vi "Features_SpecPage.vi"(10 "Spec Page Interface":T2, 11 "MetaDataObj in":refnum<class "MetaDataObj.lvclass">) -> (3 "MetaDataObj out":refnum<class "MetaDataObj.lvclass">)   [LabVIEW 2013, in "DCAFConfigurablePluginDecideFeatures.lvclass"]
uses:
  DCAFConfigurablePluginDecideFeatures.lvclass
  <resource>/dialog/NewProjectWizard/Spec Page Interface.ctl
  <resource>/dialog/NewProjectWizard/MetaDataObj/MetaDataObj.lvclass
  <vilib>/NI/Tag Bus/tag/Data Type.ctl
  <vilib>/NI/Tag Bus Module Framework/root configuration/Target Types.ctl
  <resource>/dialog/NewProjectWizard/MetaDataObj/MetaDataObj.lvclass/MetaDataObj.ctl
  DCAFConfigurablePluginDecideFeatures.lvclass/DCAFConfigurablePluginDecideFeatures.ctl
  <resource>/dialog/NewProjectWizard/MetaDataObj/Accessors/Write Project Name.vi
  Write component name.vi
  <resource>/dialog/NewProjectWizard/MetaDataObj/Accessors/Write Project Root.vi
  Write supported targets.vi
  Write supported data types.vi
  Write instances allowed.vi
  <resource>/dialog/NewProjectWizard/MetaDataObj/Accessors/Write File Prefix.vi
  <vilib>/NI/Tag Bus/tag/count types.vi
  <vilib>/NI/Tag Bus/tag/index to type.vi
  <vilib>/NI/Tag Bus Module Framework/root configuration/TBM configuration.lvclass
  <vilib>/NI/Tag Bus/tag/tag descriptor.lvclass
panel:
  in  "Tab Control":T1(tab)
  in  "Instances Allowed":i32=-1
  in  "Supported Targets":i32[](listbox)
  in  "Available Targets":i32[](listbox)
  in  "+target":bool
  in  "-target":bool
  in  "-type":bool
  in  "+type":bool
  in  "Available Data Types":i32[](listbox)
  in  "Supported Data Types":i32[](listbox)
  in  "Component Name":string
  in  "Project Root":path
  # "Execution Behaviors:"
  # "Number of classes allowed in a system. Default is infinite, -1. Examples: {PID: -1};{LED: 1}"
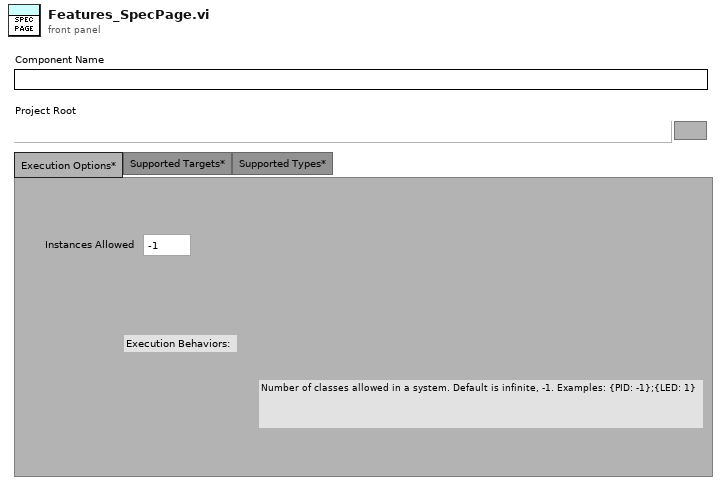
[diagram p1: front panel]
types:
  T1 = enum32{"Execution Options*", "Supported Targets*", "Supported Types*"}
  T2 = typedef "Spec Page Interface.ctl" = cluster{"\"Tab Forward To\" Refnum":refnum<vi>, "\"Tab Backward To\" Refnum":refnum<vi>, "Errors":refnum<user-event>, "Quit":refnum<user-event>}
  T3 = typedef "TBM configuration.lvclass/Target Types.ctl" = enum16{"Windows", "Mac", "Linux", "Linux RT ARM", "VxWorks", "Pharlap", "Other", "Linux RT x64"}
  T4 = typedef "tag bus.lvlib/tag descriptor.lvclass/Data Type.ctl" = enum16{"Double", "Single", "I64", "I32", "I16", "I8", "U64", "U32", "U16", "U8", "Boolean", "String", "Array of Double", "Array of Single", "Array of I64", "Array of I32", "Array of I16", "Array of I8", "Array of U64", "Array of U32", "Array of U16", "Array of U8", "Array of Boolean", "Array of String"}
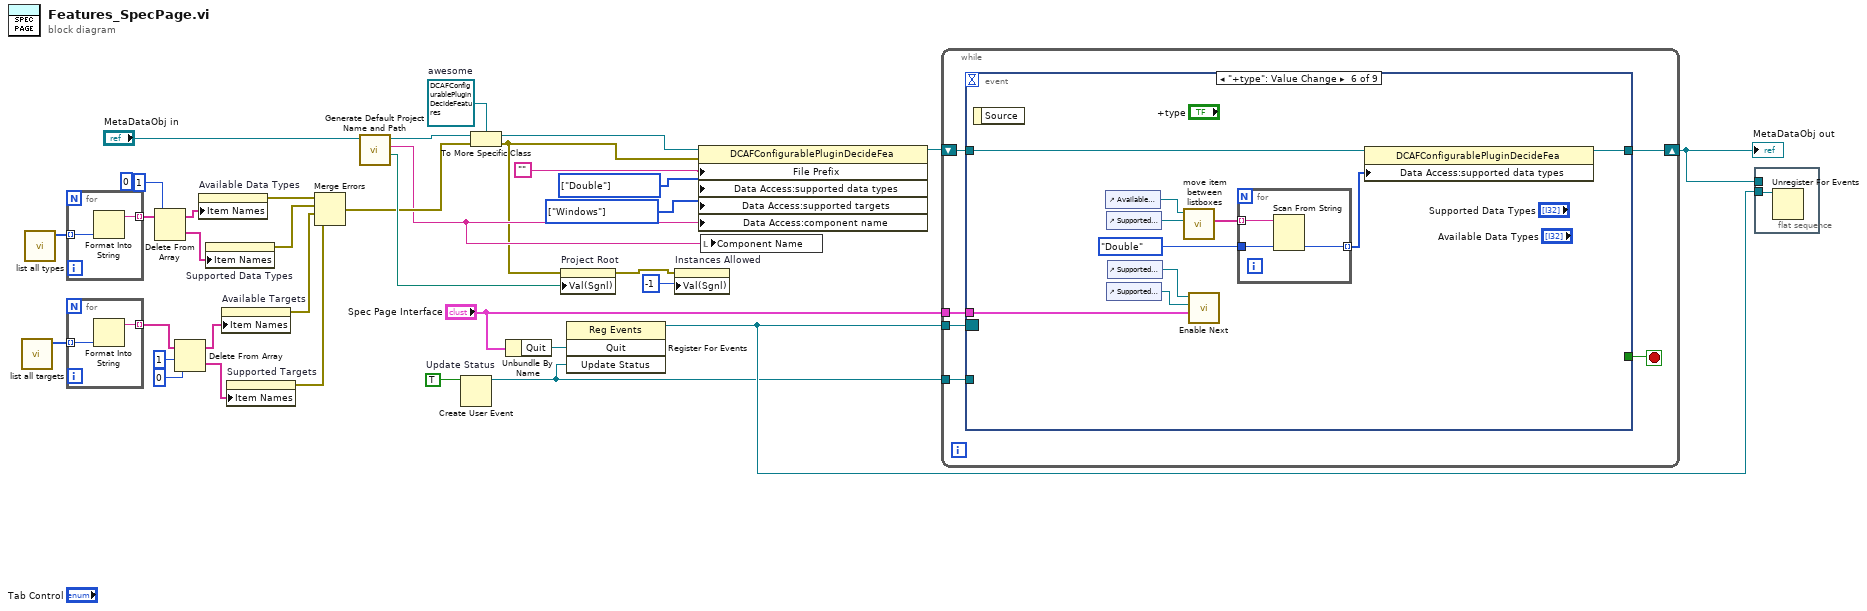
[diagram p0: block diagram]
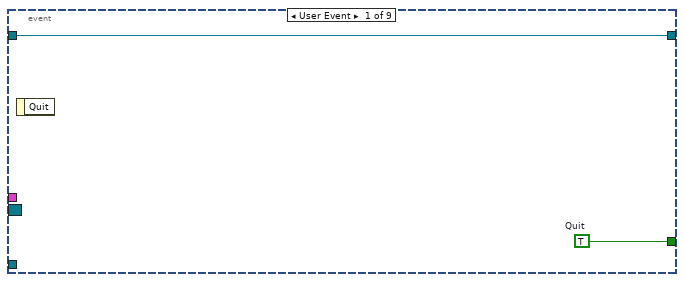
[diagram p2: hidden frame]
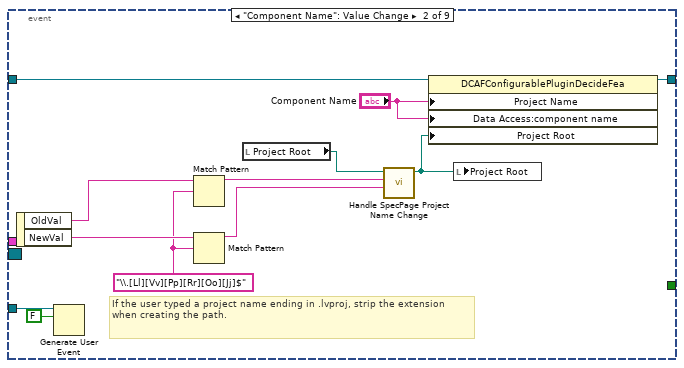
[diagram p3: hidden frame]
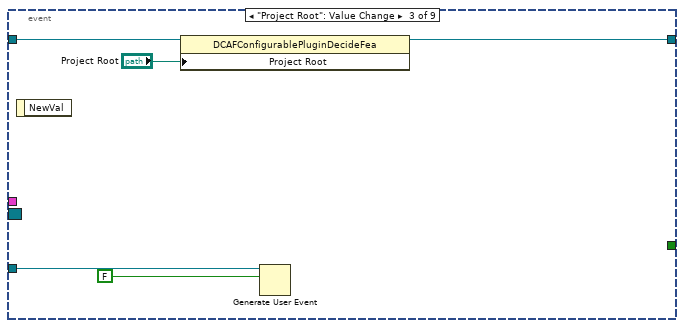
[diagram p4: hidden frame]
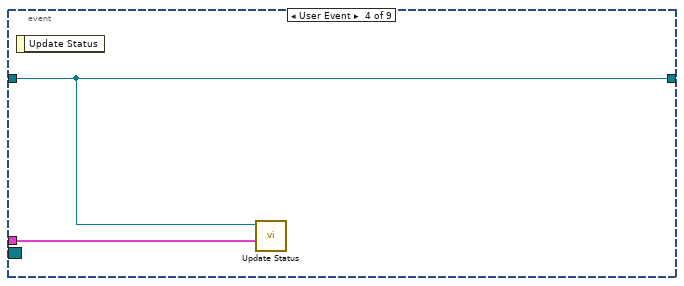
[diagram p5: hidden frame]
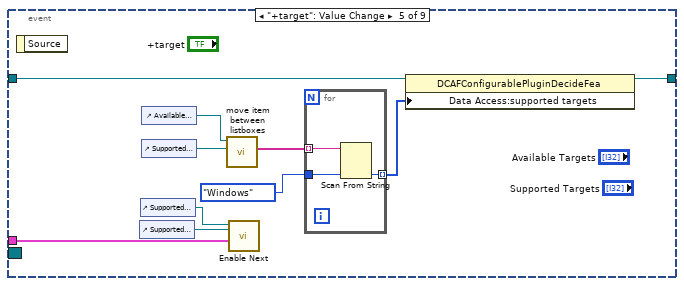
[diagram p6: hidden frame]
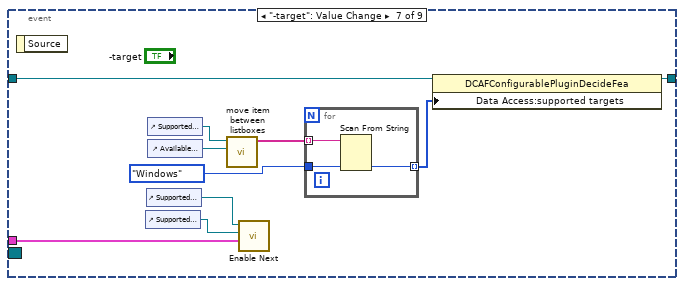
[diagram p7: hidden frame]
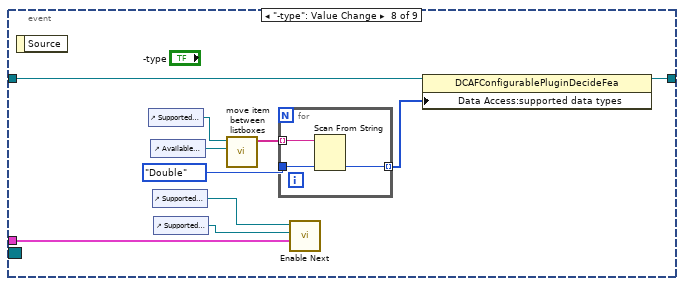
[diagram p8: hidden frame]
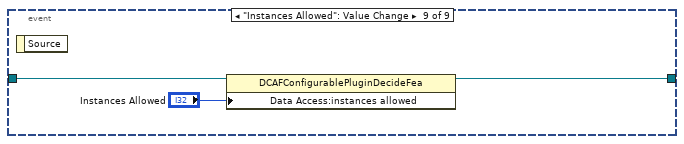
[diagram p9: hidden frame]
diagram:
  w1 = T3[] [enum."Windows"] items=["Windows", "Mac", "Linux", "Linux RT ARM", "VxWorks", "Pharlap", "Other", "Linux RT x64"] ("supported targets")
  w2 = T4[] [enum."Double"] items=["Double", "Single", "I64", "I32", "I16", "I8", "U64", "U32", "U16", "U8", "Boolean", "String", "Array of Double", "Array of Single", "Array of I64", "Array of I32", "Array of I16", "Array of I8", "Array of U64", "Array of U32", "Array of U16", "Array of U8", "Array of Boolean", "Array of String"] ("supported data types")
  w32 = TRUE  # Update Status
  w17 = refnum<class "DCAFConfigurablePluginDecideFeatures.lvclass"> refnum  # awesome
  n1 = call <vilib>:"list all targets.vi"() -> ("all targets"=w25:T3[])  [unwired: 11 in]
  n2 = call <vilib>:"list all types.vi"() -> ("all types"=w26:T4[])  [unwired: 11 in]
  n3 = for {
    tunnel: w26 -> [w38] mode=indexing
    tunnel: [w37] -> w16 mode=indexing
    n4 = Format Into String(w38) -> (resulting string=w37:string)  [unwired: 3 in, 1 out]
  }
  n5 = for {
    tunnel: w25 -> [w40] mode=indexing
    tunnel: [w39] -> w11 mode=indexing
    n6 = Format Into String(w40) -> (resulting string=w39:string)  [unwired: 3 in, 1 out]
  }
  n7 = Delete From Array(array=w16, length=1, index=0) -> (deleted portion=w14:string[], array with subset deleted=w15:string[])
  n8 = Delete From Array(array=w11, length=1, index=0) -> (deleted portion=w9:string[], array with subset deleted=w10:string[])
  n9 = property on="Available Data Types" class="LstBox (strict)"("Item Names"=w15) -> (error out=w24:errorcluster)  [unwired: 2 in, 1 out]
  n10 = property on="Supported Data Types" class="LstBox (strict)"("Item Names"=w14) -> (error out=w6:errorcluster)  [unwired: 2 in, 1 out]
  n11 = property on="Available Targets" class="LstBox (strict)"("Item Names"=w10) -> (error out=w23:errorcluster)  [unwired: 2 in, 1 out]
  n12 = property on="Supported Targets" class="LstBox (strict)"("Item Names"=w9) -> (error out=w5:errorcluster)  [unwired: 2 in, 1 out]
  n13 = Merge Errors(w24, w6, w23, w5) -> (w22:errorcluster)
  n14 = call <resource>:"Generate Default Project Name and Path.vi"("DNL_MetaDataObj in"="MetaDataObj in") -> ("Project Root"=w27:path, "Project Name"=w20:string, "DNL_MetaDataObj out"=w28:refnum<class "MetaDataObj.lvclass">)  [unwired: 8 in]
  n15 = Create User Event(user event datatype=w32) -> (user event=w30:refnum<user-event>)  [unwired: 1 in, 1 out]
  n16 = To More Specific Class(target class=w17, reference=w28, error in=w22) -> (specific class reference=w33:refnum<class "DCAFConfigurablePluginDecideFeatures.lvclass">, error out=w4:errorcluster)
  n17 = Unbundle By Name("Spec Page Interface") -> ("Quit"=w36:refnum<user-event>)
  n18 = property on="Project Root" class="Path"(error in=w4, "Val(Sgnl)"=w27) -> (error out=w3:errorcluster)  [unwired: 1 in, 1 out]
  n19 = register-events(w36, w30) -> (reference out=w35:refnum<event-registration>)  [unwired: 2 in, 1 out]
  n20 = property on="Instances Allowed" class="DigNum (strict)"(error in=w3, "Val(Sgnl)"=-1 ("Value (Signaling)")) -> ()  [unwired: 1 in, 2 out]
  n21 = property class="DCAFConfigurablePluginDecideFea"(reference=w33, error in=w4, "File Prefix"="", "Data Access:supported data types"=w2, "Data Access:supported targets"=w1, "Data Access:component name"=w20) -> (reference out=w31:refnum<class "DCAFConfigurablePluginDecideFeatures.lvclass">)  [unwired: 1 out]
  n22 = local write "Component Name"(w20) -> ()
  n23 = while {
    tunnel: "Spec Page Interface" -> [w45]
    shift-right: [w43] -> w21
    shift-left: w31 -> [w42]
    tunnel: w35 -> [w44]
    tunnel: w30 -> [w41]
    stop <- w46 stop-if-true
    n24 = event shown="[5] \"+type\": Value Change" {
      selector: w44 -> [_ _ _ _ _ _ _ _ _]
      dyn-events: _ -> [_ _ _ _ _ _ _ _ _]
      timeout: _ -> [_ _ _ _ _ _ _ _ _]
      tunnel: w45 -> [_ _ _ w66 w68 w81 w94 w107 _]
      tunnel: [w48 _ _ _ _ _ _ _ _] -> w46
      tunnel: [w47 w60 w64 w67 w76 w89 w102 w115 w121] -> w43
      tunnel: w42 -> [w47 w57 w65 w67 w77 w90 w103 w116 w122]
      tunnel: w41 -> [_ w59 w63 _ _ _ _ _ _]
      event User Event {
        w48 = TRUE  # Quit
        n25 = event-data() -> ()  [unwired: 1 in, 1 out]
      }
      event "Component Name": Value Change {
        w53 = "\\.[Ll][Vv][Pp][Rr][Oo][Jj]$" ("regular expression")
        # "If the user typed a project name ending in .lvproj, strip the extension when creating the path."
        n26 = event-data() -> ("OldVal"=w55:string, "NewVal"=w54:string)  [unwired: 1 in]
        n27 = Generate User Event(user event=w59, event data cluster=FALSE ("Update Status")) -> ()  [unwired: 2 in, 2 out]
        n28 = Match Pattern(string=w55, regular expression=w53) -> (before substring=w52:string)  [unwired: 1 in, 3 out]
        n29 = Match Pattern(string=w54, regular expression=w53) -> (before substring=w51:string)  [unwired: 1 in, 3 out]
        n30 = local read "Project Root"() -> (w56:path)
        n31 = call <resource>:"Handle SpecPage Project Name Change.vi"("Project Name New Value"=w51, "Project Name Old Value"=w52, "Project Root in"=w56) -> ("Project Root out"=w49:path)  [unwired: 8 in]
        n32 = property class="DCAFConfigurablePluginDecideFea"(reference=w57, "Project Name"="Component Name", "Data Access:component name"="Component Name", "Project Root"=w49) -> (reference out=w60:refnum<class "DCAFConfigurablePluginDecideFeatures.lvclass">)  [unwired: 1 in, 1 out]
        n33 = local write "Project Root"(w49) -> ()
      }
      event "Project Root": Value Change {
        n34 = event-data() -> ()  [unwired: 1 in, 1 out]
        n35 = property class="DCAFConfigurablePluginDecideFea"(reference=w65, "Project Root"="Project Root") -> (reference out=w64:refnum<class "DCAFConfigurablePluginDecideFeatures.lvclass">)  [unwired: 1 in, 1 out]
        n36 = Generate User Event(user event=w63, event data cluster=FALSE ("Update Status")) -> ()  [unwired: 2 in, 2 out]
      }
      event User Event {
        n37 = event-data() -> ()  [unwired: 1 in, 1 out]
        n38 = call "Update Status.vi"("Spec Page Interface"=w66, "TwoTasksMetaDataObj in"=w67) -> ()  [unwired: 10 in]
      }
      event "+target": Value Change {
        n39 = event-data() -> ()  [unwired: 1 in, 1 out]
        n40 = control-ref of="Supported Data Types"() -> (w69:refnum<vi>)
        n41 = control-ref of="Supported Targets"() -> (w70:refnum<vi>)
        n42 = control-ref of="Available Targets"() -> (w75:refnum<vi>)
        n43 = control-ref of="Supported Targets"() -> (w74:refnum<vi>)
        n44 = call "move item between listboxes.vi"("target"=w74, "source"=w75) -> ("new target"=w73:string[])  [unwired: 7 in, 2 out]
        n45 = call "Enable Next.vi"("Spec Page Interface"=w68, "Supported Data Types"=w69, "ListBox in"=w70) -> ()  [unwired: 9 in]
        n46 = for {
          tunnel: w73 -> [w80] mode=indexing
          tunnel: Target_Types."Windows" ("Target Types") -> [w79]
          tunnel: [w78] -> w71 mode=indexing
          n47 = Scan From String(input string=w80, default 1=w79) -> (output 1=w78:T3)  [unwired: 3 in, 3 out]
        }
        n48 = property class="DCAFConfigurablePluginDecideFea"(reference=w77, "Data Access:supported targets"=w71) -> (reference out=w76:refnum<class "DCAFConfigurablePluginDecideFeatures.lvclass">)  [unwired: 1 in, 1 out]
      }
      event "+type": Value Change {
        n49 = event-data() -> ()  [unwired: 1 in, 1 out]
        n50 = control-ref of="Available Data Types"() -> (w84:refnum<vi>)
        n51 = control-ref of="Supported Data Types"() -> (w86:refnum<vi>)
        n52 = control-ref of="Supported Data Types"() -> (w82:refnum<vi>)
        n53 = control-ref of="Supported Targets"() -> (w83:refnum<vi>)
        n54 = call "move item between listboxes.vi"("target"=w86, "source"=w84) -> ("new target"=w88:string[])  [unwired: 7 in, 2 out]
        n55 = call "Enable Next.vi"("Spec Page Interface"=w81, "Supported Data Types"=w82, "ListBox in"=w83) -> ()  [unwired: 9 in]
        n56 = for {
          tunnel: w88 -> [w93] mode=indexing
          tunnel: Data_Type."Double" ("Data Type") -> [w92]
          tunnel: [w91] -> w87 mode=indexing
          n57 = Scan From String(input string=w93, default 1=w92) -> (output 1=w91:T4)  [unwired: 3 in, 3 out]
        }
        n58 = property class="DCAFConfigurablePluginDecideFea"(reference=w90, "Data Access:supported data types"=w87) -> (reference out=w89:refnum<class "DCAFConfigurablePluginDecideFeatures.lvclass">)  [unwired: 1 in, 1 out]
      }
      event "-target": Value Change {
        n59 = event-data() -> ()  [unwired: 1 in, 1 out]
        n60 = control-ref of="Supported Data Types"() -> (w95:refnum<vi>)
        n61 = control-ref of="Supported Targets"() -> (w96:refnum<vi>)
        n62 = control-ref of="Supported Targets"() -> (w97:refnum<vi>)
        n63 = control-ref of="Available Targets"() -> (w99:refnum<vi>)
        n64 = call "move item between listboxes.vi"("target"=w99, "source"=w97) -> ("new source"=w98:string[])  [unwired: 7 in, 2 out]
        n65 = call "Enable Next.vi"("Spec Page Interface"=w94, "Supported Data Types"=w95, "ListBox in"=w96) -> ()  [unwired: 9 in]
        n66 = for {
          tunnel: w98 -> [w106] mode=indexing
          tunnel: Target_Types."Windows" ("Target Types") -> [w105]
          tunnel: [w104] -> w100 mode=indexing
          n67 = Scan From String(input string=w106, default 1=w105) -> (output 1=w104:T3)  [unwired: 3 in, 3 out]
        }
        n68 = property class="DCAFConfigurablePluginDecideFea"(reference=w103, "Data Access:supported targets"=w100) -> (reference out=w102:refnum<class "DCAFConfigurablePluginDecideFeatures.lvclass">)  [unwired: 1 in, 1 out]
      }
      event "-type": Value Change {
        n69 = event-data() -> ()  [unwired: 1 in, 1 out]
        n70 = control-ref of="Supported Data Types"() -> (w110:refnum<vi>)
        n71 = control-ref of="Available Data Types"() -> (w111:refnum<vi>)
        n72 = control-ref of="Supported Targets"() -> (w109:refnum<vi>)
        n73 = control-ref of="Supported Data Types"() -> (w108:refnum<vi>)
        n74 = call "move item between listboxes.vi"("target"=w111, "source"=w110) -> ("new source"=w113:string[])  [unwired: 7 in, 2 out]
        n75 = for {
          tunnel: w113 -> [w119] mode=indexing
          tunnel: Data_Type."Double" ("Data Type") -> [w118]
          tunnel: [w117] -> w114 mode=indexing
          n76 = Scan From String(input string=w119, default 1=w118) -> (output 1=w117:T4)  [unwired: 3 in, 3 out]
        }
        n77 = call "Enable Next.vi"("Spec Page Interface"=w107, "Supported Data Types"=w108, "ListBox in"=w109) -> ()  [unwired: 9 in]
        n78 = property class="DCAFConfigurablePluginDecideFea"(reference=w116, "Data Access:supported data types"=w114) -> (reference out=w115:refnum<class "DCAFConfigurablePluginDecideFeatures.lvclass">)  [unwired: 1 in, 1 out]
      }
      event "Instances Allowed": Value Change {
        n79 = event-data() -> ()  [unwired: 1 in, 1 out]
        n80 = property class="DCAFConfigurablePluginDecideFea"(reference=w122, "Data Access:instances allowed"="Instances Allowed") -> (reference out=w121:refnum<class "DCAFConfigurablePluginDecideFeatures.lvclass">)  [unwired: 1 in, 1 out]
      }
    }
  }
  "MetaDataObj out" <- w21
  n81 = flat-sequence {
    tunnel: w35 -> [w123]
    tunnel: w21 -> [_]
    frame #0 {
      n82 = Unregister For Events(event registration refnum=w123) -> ()  [unwired: 1 in, 1 out]
    }
  }
